vi "Resolve with Result.vi"(8 "error in (no error)":errorcluster, 10 "Result":variant, 11 "Result in":refnum<class "Task.lvclass">) -> (0 "error out":errorcluster)   [LabVIEW 2017, in "Futures.lvlib" / "Task.lvclass"]
uses:
  Task.lvclass
  Task.lvclass/Task.ctl
  Task Data.ctl
  Task State.ctl
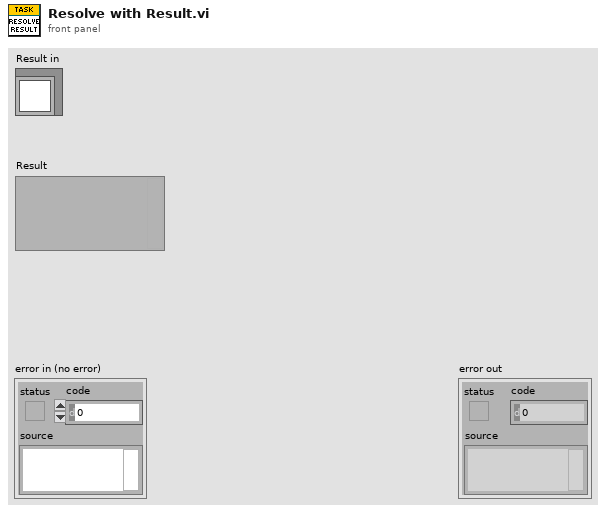
[diagram p1: front panel]
types:
  T1 = typedef "Futures.lvlib/Task.lvclass/Task State.ctl" = enum16{"Unresolved", "Ok", "Error"}
  T2 = typedef "Futures.lvlib/Task.lvclass/Task Data.ctl" = cluster{"Type":T1, "Value":variant}
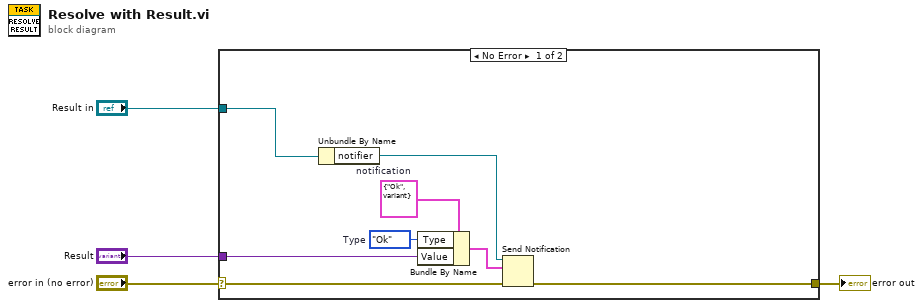
[diagram p0: block diagram]
diagram:
  n1 = case shown="No Error" "error in (no error)" {
    selector: "error in (no error)" -> [w12 w13]
    tunnel: [w11 w13] -> w3
    tunnel: "Result in" -> [w10 _]
    tunnel: "Result" -> [w5 _]
    frame No Error {
      w6 = Task_State."Ok"  # Type
      w8 = T2 {"Type"=enum."Ok", "Value"=variant}  # notification
      n2 = Unbundle By Name(w10) -> ("notifier"=w9:refnum<notifier>)
      n3 = Bundle By Name(cluster=w8, "Type"=w6, "Value"=w5) -> (w7:T2)
      n4 = Send Notification(notification=w7, notifier=w9, error in (no error)=w12) -> (error out=w11:errorcluster)  [unwired: 1 out]
    }
    frame Error {
    }
  }
  "error out" <- w3
